vi "Sonic Systems P100 Test Program 2.vi"() -> ()   [LabVIEW 2018, in "Sonic Systems P100.lvlib"]
uses:
  Sonic Systems P100.lvlib
  Sonic Systems P100 Settings.ctl
panel:
  out "Power":i32
  out "Connection Error":bool
  out "Running":bool
  out "Amplitude":i32
  in  "stop":bool
  in  "Setpoint":dbl min=0.0 max=16.0 step=0.5 format="%04.1f"
  in  "Pause":bool
  out "SS P100 Settings Out":T1
  out "error out":errorcluster
  in  "error in (no error)":errorcluster
  in  "SS P100 Settings":T1
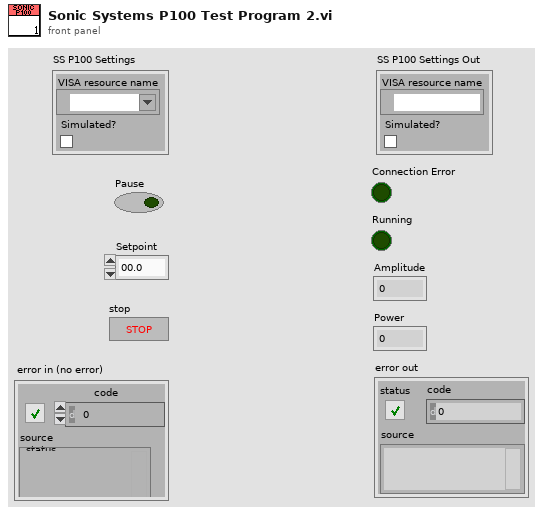
[diagram p1: front panel]
types:
  T1 = typedef "Sonic Systems P100.lvlib/Sonic Systems P100 Settings.ctl" = cluster{"VISA resource name":refnum<visa-resource-name>, "Simulated?":bool}
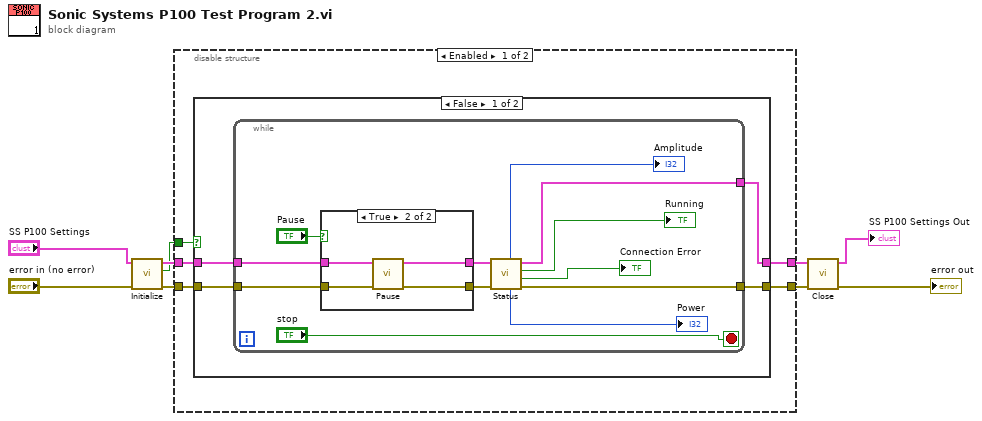
[diagram p0: block diagram]
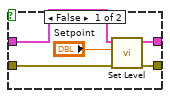
[diagram p2: hidden frame]
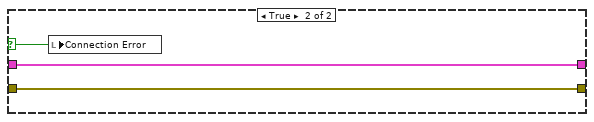
[diagram p3: hidden frame]
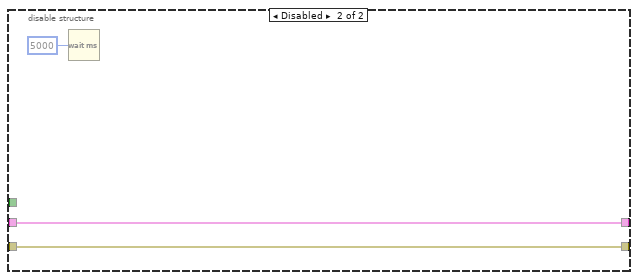
[diagram p4: hidden frame]
diagram:
  n1 = call "Initialize.vi"("error in (no error)"="error in (no error)", "SS P100 Settings"="SS P100 Settings") -> ("error out"=w6:errorcluster, "Connection Error"=w5:bool, "SS P100 Settings"=w7:T1)  [unwired: 7 in]
  n2 = disable-structure shown="Enabled" {
    disable-tunnel: w7 -> [w14 w45]
    disable-tunnel: w6 -> [w13 w44]
    disable-tunnel: w5 -> [w12 _]
    disable-tunnel: [w11 w44] -> w4
    disable-tunnel: [w10 w45] -> w3
    frame Enabled {
      n3 = case shown="False" w12 {
        selector: w12 -> [_ w40]
        tunnel: w14 -> [w18 w42]
        tunnel: w13 -> [w17 w41]
        tunnel: [w16 w41] -> w11
        tunnel: [w15 w42] -> w10
        frame False {
          n4 = while {
            tunnel: w18 -> [w30]
            tunnel: w17 -> [w29]
            tunnel: [w26] -> w15
            tunnel: [w25] -> w16
            stop <- "stop" stop-if-true
            n5 = case shown="True" "Pause" {
              tunnel: w30 -> [w35 w39]
              tunnel: w29 -> [w34 w38]
              tunnel: [w33 w37] -> w28
              tunnel: [w32 w36] -> w27
              frame False {
                n6 = call "Set Level.vi"("error in (no error)"=w34, "Setpoint"="Setpoint", "SS P100 Settings In"=w35) -> ("error out"=w33:errorcluster, "SS P100 Settings Out"=w32:T1)  [unwired: 6 in, 1 out]
              }
              frame True {
                n7 = call "Pause.vi"("error in (no error)"=w38, "SS P100 Settings In"=w39) -> ("error out"=w37:errorcluster, "SS P100 Settings Out"=w36:T1)  [unwired: 8 in]
              }
            }
            n8 = call "Status.vi"("error in (no error)"=w28, "SS P100 Settings In"=w27) -> ("error out"=w25:errorcluster, "Connection Error"=→"Connection Error":bool, "Running"=→"Running":bool, "SS P100 Settings Out"=w26:T1, "Power"=→"Power":i32, "Amplitude"=→"Amplitude":i32)  [unwired: 4 in]
          }
        }
        frame True {
          n9 = local write "Connection Error"(w40) -> ()
        }
      }
    }
    frame Disabled {
      n10 = Wait (ms)(milliseconds to wait=u32 5000) -> ()  [unwired: 1 out]
    }
  }
  n11 = call "Close.vi"("error in (no error)"=w4, "SS P100 Settings"=w3) -> ("error out"=→"error out":errorcluster, "SS P100 Settings"=→"SS P100 Settings Out":T1)  [unwired: 8 in]
